vi "Octave Display (line+cursor).vi"(1 "bandedge frequencies [Hz]":T1(array[cluster]) {"midband" format="%.2f"; "f high" format="%.2f"; "f low" format="%.2f"}, 2 "nominal frequencies [Hz]":dbl[](array[numeric]) format="%.2f", 3 "band power [dB EU]":dbl[](array[numeric]) format="%.2f") -> (0 "octave display":cluster{dbl[], dbl[]}[](array[cluster]) {"?" format="%.2f"; "?" format="%.2f"})   [LabVIEW 2017]
doc: "Converts the results of any fractional-octave analysis into an octave spectrum to display as a line graph. Use this VI to display multiple octave spectra on the same graph. This VI generates two plots for each fractional-octave result. The second plot is used to lock a cursor to the center frequencies."
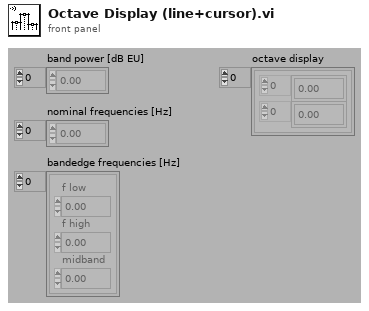
[diagram p1: front panel]
types:
  T1 = cluster{"f low":dbl, "f high":dbl, "midband":dbl}[]
  T2 = cluster{"nominal frequencies [Hz]":dbl[], "band power [dB EU]":dbl[]}
  T3 = cluster{"nominal frequencies [Hz]":dbl[], "band power [dB EU]":dbl[]}[]
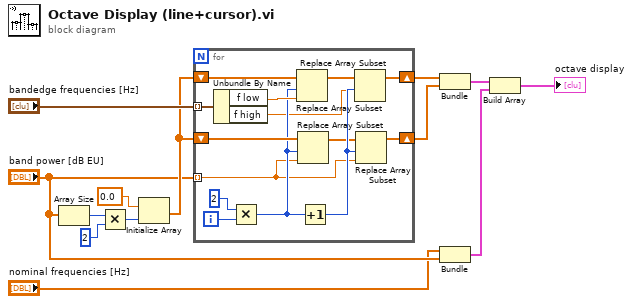
[diagram p0: block diagram]
diagram:
  n1 = Array Size(array="band power [dB EU]") -> (size(s)=w10:i32)
  n2 = Multiply(x=w10, y=2) -> (x*y=w8:i32)
  n3 = Initialize Array(0.0, w8) -> (w6:dbl[])
  n4 = for {
    tunnel: "bandedge frequencies [Hz]" -> [w27] mode=indexing
    tunnel: "band power [dB EU]" -> [w17] mode=indexing
    shift-right: [w15] -> w12
    shift-left: w6 -> [w24]
    shift-right: [w14] -> w11
    shift-left: w6 -> [w21]
    i -> [w26]
    n5 = Unbundle By Name(w27) -> ("f low"=w23:dbl, "f high"=w16:dbl)
    n6 = Multiply(x=2, y=w26) -> (x*y=w20:i32)
    n7 = Replace Array Subset(array=w24, new element=w23, index=w20) -> (w22:dbl[])
    n8 = Replace Array Subset(array=w21, new element=w17, index=w20) -> (w18:dbl[])
    n9 = Increment(x=w20) -> (x+1=w19:i32)
    n10 = Replace Array Subset(array=w22, new element=w16, index=w19) -> (w15:dbl[])
    n11 = Replace Array Subset(array=w18, new element=w17, index=w19) -> (w14:dbl[])
  }
  n12 = Bundle(w12, w11) -> (w3:cluster{dbl[], dbl[]})  [unwired: 1 in]
  n13 = Bundle("nominal frequencies [Hz]"="nominal frequencies [Hz]", "band power [dB EU]"="band power [dB EU]") -> (w2:T2)  [unwired: 1 in]
  n14 = Build Array(w3, w2) -> (→"octave display":T3)
